vi "target.vi"() -> ()   [LabVIEW 2020]
uses:
  <vilib>/Analysis/Matrix/Numeric/Conversions/Array To Matrix - RA.vi
  <vilib>/Analysis/Matrix/Numeric/Conversions/Array To Matrix - RA2.vi
  <vilib>/Analysis/Matrix/Numeric/Conversions/Matrix To Array - RM.vi
  <vilib>/Analysis/Matrix/NI_Matrix.lvlib
panel:
  out "loop timing":dbl
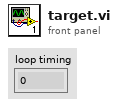
[diagram p1: front panel]
types:
  T1 = typedef "NI_Matrix.lvlib/RealMatrix.ctl" = dbl[][]
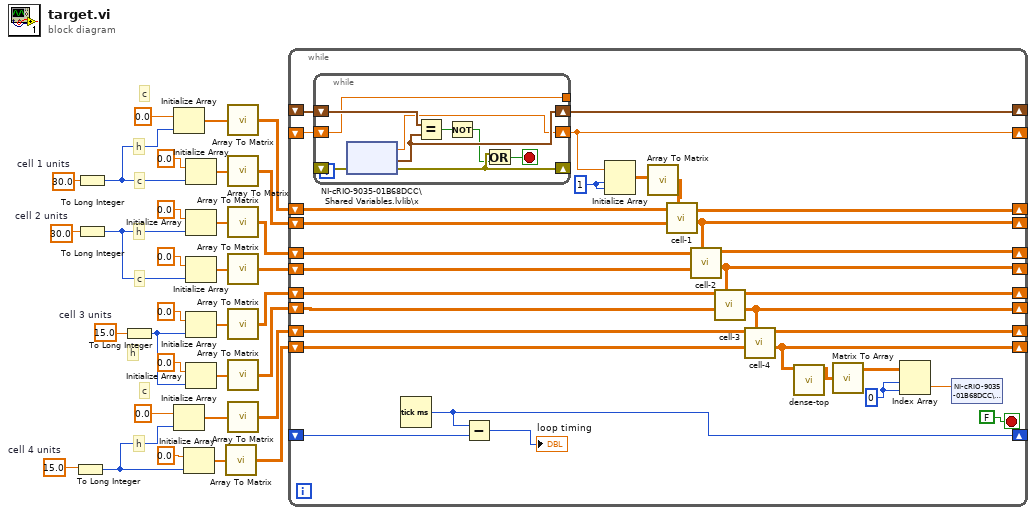
[diagram p0: block diagram]
diagram:
  w22 = 15.0  # cell 4 units
  w25 = 15.0  # cell 3 units
  w28 = 30.0  # cell 2 units
  w31 = 30.0  # cell 1 units
  # "c"
  # "c"
  # "c"
  # "c"
  # "h"
  # "h"
  # "h"
  # "h"
  n1 = To Long Integer(number=w22) -> (32bit integer=w9:i32)
  n2 = To Long Integer(number=w31) -> (32bit integer=w18:i32)
  n3 = To Long Integer(number=w28) -> (32bit integer=w15:i32)
  n4 = To Long Integer(number=w25) -> (32bit integer=w12:i32)
  n5 = Initialize Array(0.0, w18) -> (w19:dbl[])
  n6 = Initialize Array(0.0, w9) -> (w10:dbl[])
  n7 = Initialize Array(0.0, w9) -> (w21:dbl[])
  n8 = Initialize Array(0.0, w18) -> (w30:dbl[])
  n9 = Initialize Array(0.0, w15) -> (w16:dbl[])
  n10 = Initialize Array(0.0, w15) -> (w27:dbl[])
  n11 = Initialize Array(0.0, w12) -> (w13:dbl[])
  n12 = Initialize Array(0.0, w12) -> (w24:dbl[])
  n13 = call-poly <vilib>:"Array To Matrix.vi"("Real 1D Array"=w21) -> ("Real Matrix (Column Vector)"=w1:T1)
  n14 = call-poly <vilib>:"Array To Matrix.vi"("Real 1D Array"=w19) -> ("Real Matrix (Column Vector)"=w8:T1)
  n15 = call-poly <vilib>:"Array To Matrix.vi"("Real 1D Array"=w30) -> ("Real Matrix (Column Vector)"=w7:T1)
  n16 = call-poly <vilib>:"Array To Matrix.vi"("Real 1D Array"=w16) -> ("Real Matrix (Column Vector)"=w6:T1)
  n17 = call-poly <vilib>:"Array To Matrix.vi"("Real 1D Array"=w27) -> ("Real Matrix (Column Vector)"=w5:T1)
  n18 = call-poly <vilib>:"Array To Matrix.vi"("Real 1D Array"=w13) -> ("Real Matrix (Column Vector)"=w4:T1)
  n19 = call-poly <vilib>:"Array To Matrix.vi"("Real 1D Array"=w24) -> ("Real Matrix (Column Vector)"=w3:T1)
  n20 = call-poly <vilib>:"Array To Matrix.vi"("Real 1D Array"=w10) -> ("Real Matrix (Column Vector)"=w2:T1)
  n21 = while {
    shift-right: [w49] -> _
    shift-left: w8 -> [w63]
    shift-right: [w50] -> _
    shift-left: w7 -> [w62]
    shift-right: [w47] -> _
    shift-left: w6 -> [w61]
    shift-right: [w48] -> _
    shift-left: w5 -> [w60]
    shift-right: [w45] -> _
    shift-left: w4 -> [w59]
    shift-right: [w46] -> _
    shift-left: w3 -> [w58]
    shift-right: [w44] -> _
    shift-left: w2 -> [w57]
    shift-right: [w41] -> _
    shift-left: w1 -> [w56]
    shift-right: [w52] -> _
    shift-left: _ -> [w55]
    shift-right: [w54] -> _
    shift-left: _ -> [w53]
    shift-right: [w35] -> _
    shift-left: _ -> [w33]
    stop <- FALSE stop-if-true
    w39 = 0
    w51 = 1
    n22 = while {
      shift-right: [w71] -> w54
      shift-left: w53 -> [w70]
      shift-right: [w69] -> _
      shift-left: _ -> [w72]
      shift-right: [w64] -> w52
      shift-left: w55 -> [w65]
      tunnel: [w65] -> _
      stop <- w67 stop-if-true
      n23 = shared-variable "NI-cRIO-9035-01B68DCC\\Shared Variables.lvlib\\x"(error in=w72) -> (w64:dbl, error out=w69:errorcluster, w71:timestamp)
      n24 = Equal?(x=w70, y=w71) -> (x = y?=w66:bool)
      n25 = Not(x=w66) -> (.not. x?=w68:bool)
      n26 = Or(x=w69, y=w68) -> (x .or. y?=w67:bool)
    }
    n27 = Tick Count (ms)() -> (millisecond timer value=w35:u32)
    n28 = Subtract(x=w35, y=w33) -> (x-y=→"loop timing":u32)
    n29 = Initialize Array(w52, w51, w51) -> (w43:dbl[][])
    n30 = call-poly <vilib>:"Array To Matrix.vi"("Real 2D Array"=w43) -> ("Real Matrix"=w42:T1)
    n31 = call "cell-1.vi"("x"=w42, "h"=w62, "c"=w63) -> ("h + 1"=w50:T1, "c + 1"=w49:T1)  [unwired: 7 in]
    n32 = call "cell-2.vi"("x"=w50, "h"=w60, "c"=w61) -> ("h + 1"=w48:T1, "c + 1"=w47:T1)  [unwired: 7 in]
    n33 = call "cell-3.vi"("x"=w48, "h"=w58, "c"=w59) -> ("h + 1"=w46:T1, "c + 1"=w45:T1)  [unwired: 7 in]
    n34 = call "cell-4.vi"("x"=w46, "h"=w56, "c"=w57) -> ("h + 1"=w41:T1, "c + 1"=w44:T1)  [unwired: 7 in]
    n35 = call "dense-top.vi"("x_dense"=w41) -> ("y_out"=w38:T1)  [unwired: 10 in]
    n36 = call-poly <vilib>:"Matrix To Array.vi"("Real Matrix"=w38) -> ("Real 2D Array"=w40:dbl[][])
    n37 = Index Array(array=w40, index (row)=w39, index (col)=w39) -> (element=w37:dbl)
    n38 = shared-variable "NI-cRIO-9035-01B68DCC\\Shared Variables.lvlib\\y"(w37) -> ()  [unwired: 1 in, 1 out]
  }
